vi "Get Module Config.vi"(8 "error in (no error)":errorcluster, 11 "9224 in":refnum<class "9224.lvclass">) -> (0 "error out":errorcluster, 2 "Config Channels":dbl[](array[numeric]), 3 "9224 out":refnum<class "9224.lvclass">)   [LabVIEW 2017, in "Modules.lvlib" / "9224.lvclass"]
uses:
  9224.lvclass
  RSI Module/RSI Module.lvclass
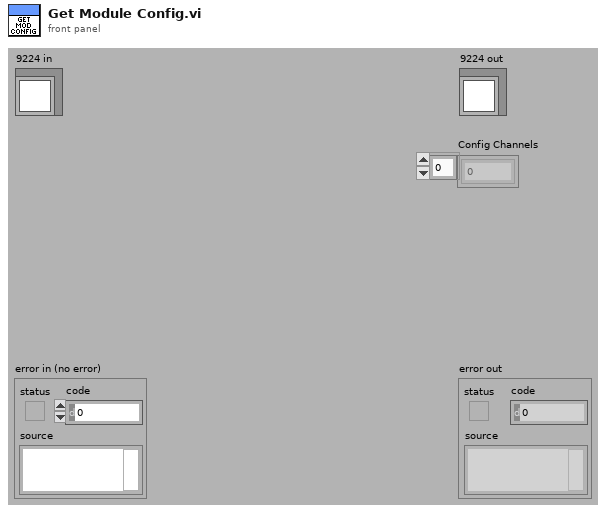
[diagram p1: front panel]
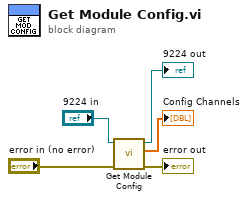
[diagram p0: block diagram]
diagram:
  n1 = call-parent "Get Module Config.vi"("error in (no error)"="error in (no error)", "RSI Module in"="9224 in") -> ("error out"=→"error out":errorcluster, "Config Channels"=→"Config Channels":dbl[], "RSI Module out"=→"9224 out":refnum<class "9224.lvclass">)  [unwired: 7 in]
